vi "Compressor Loop.vi"(0 "error in (no error)":errorcluster) -> ()   [LabVIEW 2011]
uses:
  <vilib>/Rock Robotics/WPI/Relay/WPI_RelayValue.ctl
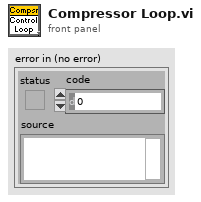
[diagram p1: front panel]
types:
  T1 = typedef "WPI_DigitalInputDevRef.ctl" = cluster{"DevStatus":errorcluster, "DIO Channel":T2, "Digital Module":T3}
  T2 = typedef "FPGA_DIOChannel.ctl" = enum8{"DIO 1", "DIO 2", "DIO 3", "DIO 4", "DIO 5", "DIO 6", "DIO 7", "DIO 8", "DIO 9", "DIO 10", "DIO 11", "DIO 12", "DIO 13", "DIO 14", "Invalid"}
  T3 = typedef "FPGA_TypedefDigitalModule.ctl" = enum16{"Digital Module 1", "Digital Module 2"}
  T4 = typedef "WPI_RelayDevRef.ctl" = cluster{"DevStatus":errorcluster, "Relay Channel":T5, "Digital Module":T3, "Relay Direction":T6}
  T5 = typedef "FPGA_DIORelayChannel.ctl" = enum8{"Relay 1", "Relay 2", "Relay 3", "Relay 4", "Relay 5", "Relay 6", "Relay 7", "Relay 8", "Invalid"}
  T6 = typedef "WPI_RelayDirection.ctl" = enum16{"Both directions", "Forward only", "Reverse only"}
  T7 = typedef "WPI_RelayValue.ctl" = enum16{"Off", "On", "Forward", "Reverse"}
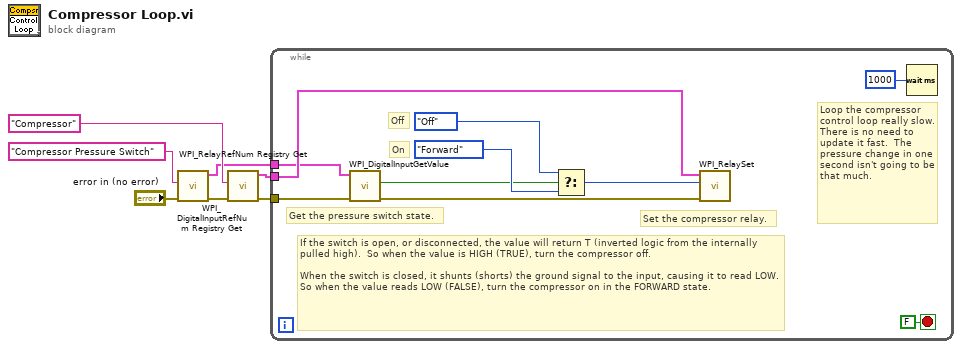
[diagram p0: block diagram]
diagram:
  n1 = call <vilib>:"WPI_DigitalInputRefNum Registry Get.vi"("error in (no error)"="error in (no error)", "refnum name"="Compressor Pressure Switch") -> ("error out"=w3:errorcluster, "DigitalInputDevRef"=w4:T1)  [unwired: 8 in]
  n2 = call <vilib>:"WPI_RelayRefNum Registry Get.vi"("error in (no error)"=w3, "refnum name"="Compressor") -> ("error out"=w2:errorcluster, "RelayDevRef"=w1:T4)  [unwired: 8 in]
  n3 = while {
    tunnel: w1 -> [w15]
    tunnel: w2 -> [w14]
    tunnel: w4 -> [w8]
    stop <- FALSE stop-if-true
    # "On"
    # "Off"
    # "Loop the compressor control loop really slow.  There is no need to update it fast.  The pressure change in one second isn't going to be that much."
    # "If the switch is open, or disconnected, the value will return T (inverted logic from the internally pulled high).  So when the value is HIGH (TRUE), turn the compressor off.\n\nWhen the switch is closed, it shunts (shorts) the ground signal to the input, causing it to read LOW.  So when the value reads LOW (FALSE), turn the compressor on in the FORWARD state."
    # "Set the compressor relay."
    # "Get the pressure switch state."
    n4 = call <vilib>:"WPI_DigitalInputGetValue.vi"("error in (no error)"=w14, "DigitalInputDevRef"=w8) -> ("error out"=w13:errorcluster, "Value"=w10:bool)  [unwired: 7 in, 1 out]
    n5 = Select(t=WPI_RelayValue."Off" ("RelayValue"), s=w10, f=WPI_RelayValue."Forward" ("RelayValue")) -> (s? t:f=w9:T7)
    n6 = call <vilib>:"WPI_RelaySet.vi"("error in (no error)"=w13, "RelayValue"=w9, "RelayDevRef"=w15) -> ()  [unwired: 7 in, 2 out]
    n7 = Wait (ms)(milliseconds to wait=u32 1000) -> ()  [unwired: 1 out]
  }
